vi "Get Dichotomie.vi"(11 "Collision in":refnum<class "Collision.lvclass">) -> (2 "Dichotomie out":i32)   [LabVIEW 2024, in "Collision.lvclass"]
doc: "MIT Licence\nCopyright (c) 2024 David Grollier"
uses:
  Collision.lvclass
  Collision.lvclass/Collision.ctl
  Game Componants/Game Board Component/Movable/Movable.lvclass
  Game Componants/Game Board Component/Movable/Movable.lvclass/Movable.ctl
  Game Componants/Game Componants.lvclass/Game Componants.ctl
  Game Componants/Game Componants.lvclass
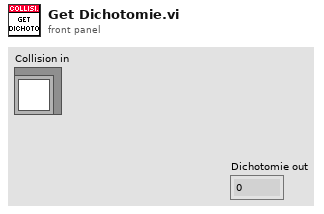
[diagram p1: front panel]
types:
  T1 = typedef "Coordinates.ctl" = cluster{"x":dbl, "y":dbl}
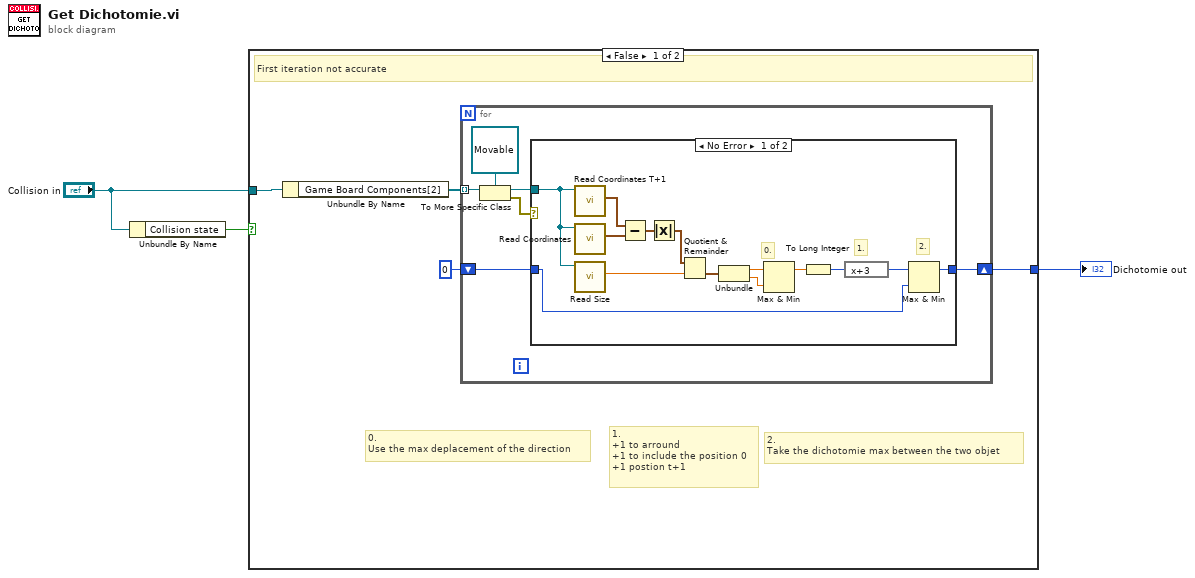
[diagram p0: block diagram]
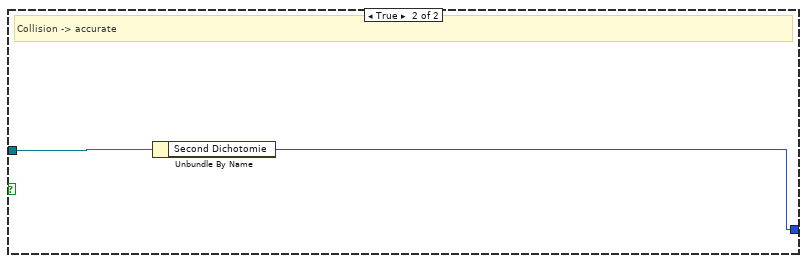
[diagram p3: hidden frame]
diagram:
  n1 = Unbundle By Name("Collision in") -> ("Collision state"=w1:bool)
  n2 = case shown="False" w1 {
    tunnel: [w7 w29] -> w3
    tunnel: "Collision in" -> [w4 w30]
    frame False {
      # "0.\nUse the max deplacement of the direction"
      # "2.\nTake the dichotomie max between the two objet"
      # "1.\n+1 to arround\n+1 to include the position 0\n+1 postion t+1"
      # "First iteration not accurate"
      n3 = Unbundle By Name(w4) -> ("Game Board Components[2]"=w6:refnum<class "Game Board Component.lvclass">[])
      n4 = for {
        tunnel: w6 -> [w12] mode=indexing
        shift-right: [w9] -> w7
        shift-left: 0 -> [w10]
        n5 = To More Specific Class(target class=refnum<class "Movable.lvclass"> refnum ("Movable.lvclass"), reference=w12) -> (specific class reference=w11:refnum<class "Movable.lvclass">, error out=w8:errorcluster)  [unwired: 1 in]
        n6 = case shown="No Error" w8 {
          tunnel: w11 -> [w27 _]
          tunnel: w10 -> [w16 w28]
          tunnel: [w15 w28] -> w9
          frame No Error {
            # "0."
            # "2."
            # "1."
            n7 = call "Read Coordinates T+1.vi"("Movable in"=w27) -> ("Coordinates"=w26:T1)  [unwired: 10 in]
            n8 = call "Read Coordinates.vi"("Game Componants in"=w27) -> ("Coordinates"=w25:T1)  [unwired: 10 in]
            n9 = call "Read Size.vi"("Movable in"=w27) -> ("Size"=w22:dbl)  [unwired: 10 in]
            n10 = Subtract(x=w26, y=w25) -> (x-y=w24:T1)
            n11 = Absolute Value(x=w24) -> (abs(x)=w23:T1)
            n12 = Quotient & Remainder(x=w23, y=w22) -> (floor(x/y)=w18:T1)  [unwired: 1 out]
            n13 = Unbundle(w18) -> ("x"=w19:dbl, "y"=w20:dbl)
            n14 = Max & Min(x=w19, y=w20) -> (max(x,y)=w21:dbl)  [unwired: 1 out]
            n15 = To Long Integer(number=w21) -> (32bit integer=w14:i32)
            n16 = expression code="x+3"(w14) -> (w17:i32)
            n17 = Max & Min(x=w17, y=w16) -> (max(x,y)=w15:i32)  [unwired: 1 out]
          }
          frame Error {
            # "Not a movable : doesn't move"
          }
        }
      }
    }
    frame True {
      # "Collision -> accurate"
      n18 = Unbundle By Name(w30) -> ("Second Dichotomie"=w29:i32)
    }
  }
  "Dichotomie out" <- w3
